vi "Get YArrayType.vi"(8 "error in (no error)":errorcluster, 11 "LVAnalogWaveformType.lvclass in":refnum<class "LVAnalogWaveformType.lvclass">) -> (0 "error out":errorcluster, 2 "YArrayType":refnum<class "LVType.lvclass">, 3 "LVAnalogWaveformType.lvclass out":refnum<class "LVAnalogWaveformType.lvclass">)   [LabVIEW 2020, in "LVDataTypes.lvlib" / "LVAnalogWaveformType.lvclass"]
uses:
  <vilib>/AppBuilder/Engine/WebServiceDescription/LVDataTypes/LVAnalogWaveformType/LVAnalogWaveformType.lvclass
  <vilib>/AppBuilder/Engine/WebServiceDescription/LVDataTypes/LVType/LVType.lvclass
  <vilib>/AppBuilder/Engine/WebServiceDescription/LVDataTypes/LVAnalogWaveformType/LVAnalogWaveformType.lvclass/LVAnalogWaveformType.ctl
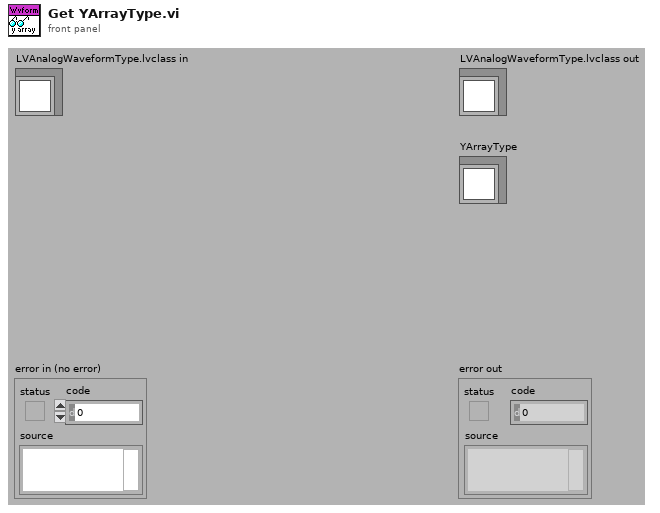
[diagram p1: front panel]
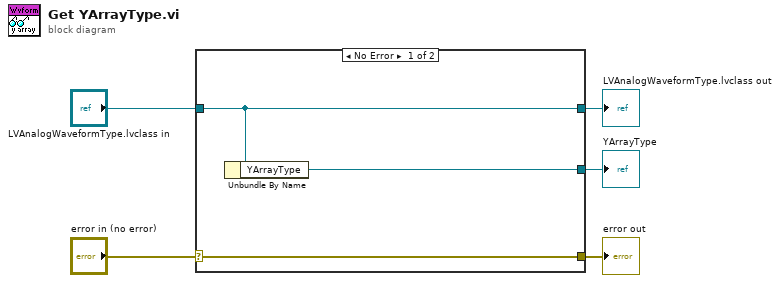
[diagram p0: block diagram]
diagram:
  n1 = case shown="No Error" "error in (no error)" {
    selector: "error in (no error)" -> [w8 w9]
    tunnel: [w8 w9] -> w4
    tunnel: [w7 w10] -> w2
    tunnel: "LVAnalogWaveformType.lvclass in" -> [w7 w10]
    tunnel: [w6 _] -> w1
    frame No Error {
      n2 = Unbundle By Name(w7) -> ("YArrayType"=w6:refnum<class "LVType.lvclass">)
    }
    frame Error {
    }
  }
  "error out" <- w4
  "LVAnalogWaveformType.lvclass out" <- w2
  "YArrayType" <- w1
